vi "CuLab_Tensor_to_SpecWF.vi"(7 "dt":dbl, 11 "Y":sgl[](array[numeric])) -> (3 "Spectrum WF":waveform(sgl))   [LabVIEW 2020]
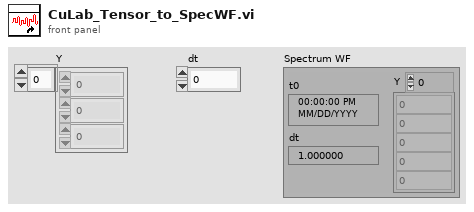
[diagram p1: front panel]
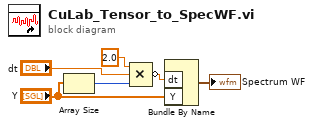
[diagram p0: block diagram]
diagram:
  n1 = Array Size(array="Y") -> (size(s)=w4:i32)
  n2 = Compound Arithmetic op=MULTIPLY(2.0 ("y"), "dt", w4) -> (invert w3:dbl)
  n3 = Bundle By Name("dt"=w3, "Y"="Y") -> (→"Spectrum WF":waveform(sgl))  [unwired: 1 in]
